vi "Build Tree.vi"(5 "Defer Updates (T)":bool=TRUE, 7 "Tree":refnum<vi>, 8 "error in (no error)":errorcluster, 11 "Tree Map in":refnum<class "Tree Map.lvclass">) -> (0 "error out":errorcluster, 3 "Tree Map out":refnum<class "Tree Map.lvclass">)   [LabVIEW 2020, in "Tree Map.lvlib" / "Tree Map.lvclass"]
uses:
  Tree Map.lvclass
  Tree Map.lvclass/Tree Map.ctl
  Tree Map.lvlib
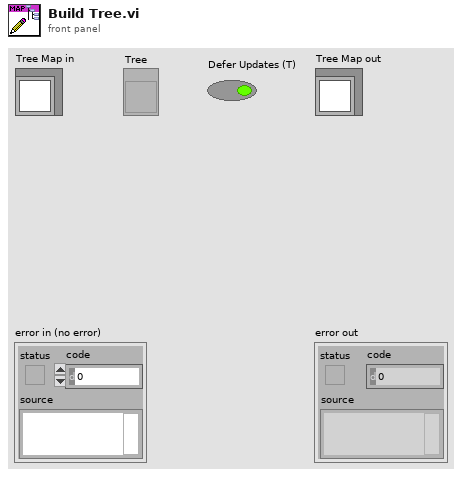
[diagram p1: front panel]
types:
  T1 = typedef "LVNodeAndColumnTypeDef.ctl" = cluster{"Node":string, "Column":i32}
  T2 = typedef "Tree Map.lvlib/Tree Map.lvclass/Tree Entry.ctl" = cluster{"Hierarchy":string[], "Name":string, "Columns":string[], "Leaf":bool, "Extra":T3}
  T3 = typedef "Tree Map.lvlib/Tree Map.lvclass/Extra Entry Info.ctl" = cluster{"BG Color":u32, "Symbol":i32}
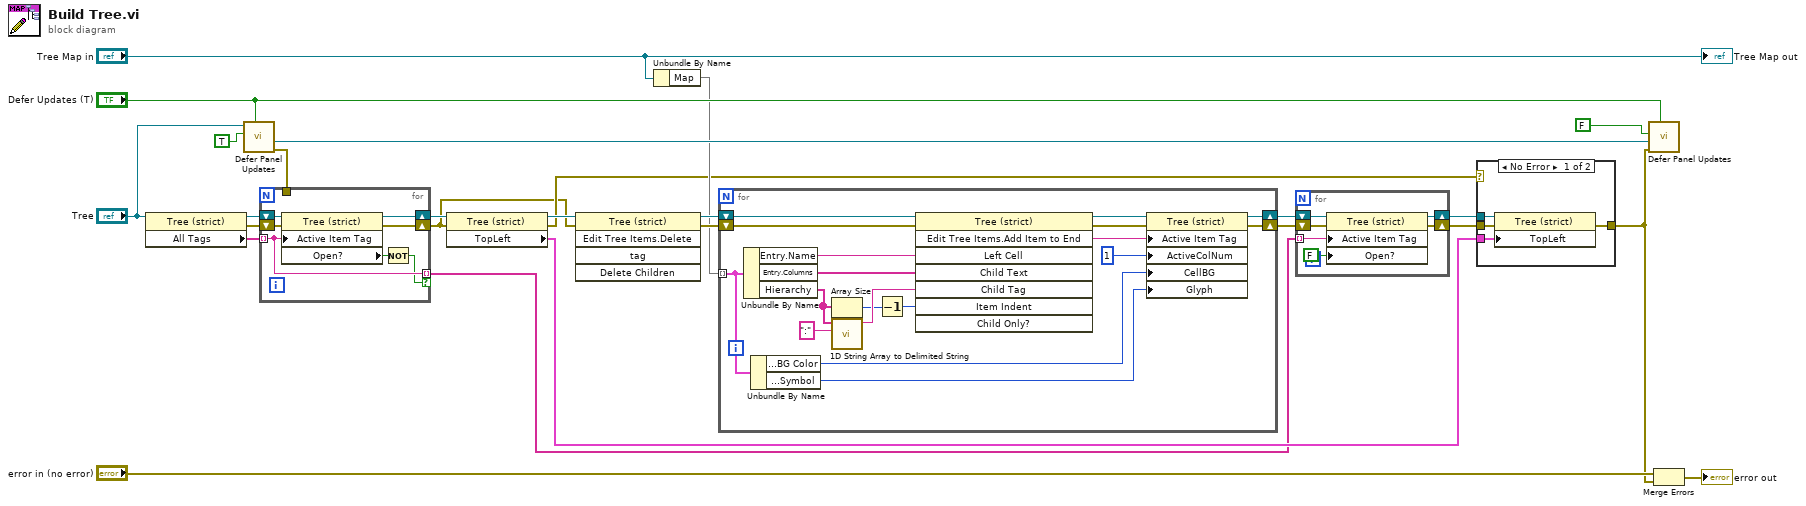
[diagram p0: block diagram]
diagram:
  n1 = property class="Tree (strict)"(reference="Tree") -> (reference out=w20:refnum<vi>, error out=w7:errorcluster, "All Tags"=w21:string[])  [unwired: 1 in]
  n2 = call "Defer Panel Updates.vi"("Set Defer (T)"="Defer Updates (T)", "Defer"=TRUE, "Tree (Front Panel)"="Tree") -> ("error out"=w8:errorcluster, "Front Panel"=w12:refnum<vi>)  [unwired: 7 in]
  n3 = for {
    tunnel: w21 -> [w31] mode=indexing
    shift-right: [w29] -> w19
    shift-left: w20 -> [w33]
    tunnel: [w31] -> w18 mode=indexing if=w30
    tunnel: w8 -> [_]
    shift-right: [w27] -> w1
    shift-left: w7 -> [w28]
    n4 = property class="Tree (strict)"(reference=w33, error in=w28, "Active Item Tag"=w31) -> (reference out=w29:refnum<vi>, error out=w27:errorcluster, "Open?"=w32:bool)
    n5 = Not(x=w32) -> (.not. x?=w30:bool)
  }
  n6 = property class="Tree (strict)"(reference=w19, error in=w1) -> (reference out=w23:refnum<vi>, error out=w2:errorcluster, "TopLeft"=w22:T1)
  n7 = invoke class="Tree (strict)" method="Edit Tree Items.Delete"(reference=w23, error in=w1) -> (reference out=w24:refnum<vi>, error out=w26:errorcluster)  [unwired: 3 in, 3 out]
  n8 = Unbundle By Name("Tree Map in") -> ("Map"=w9:map{string[], T2})
  n9 = for {
    shift-right: [w37] -> w16
    shift-left: w24 -> [w51]
    tunnel: w9 -> [w42] mode=indexing
    shift-right: [w36] -> w6
    shift-left: w26 -> [w44]
    n10 = Unbundle By Name(w42) -> ("Entry.Name"=w45:string, "Entry.Columns"=w46:string[], "Hierarchy"=w43:string[])
    n11 = Unbundle By Name(w42) -> ("Entry.Extra.BG Color"=w35:u32, "Entry.Extra.Symbol"=w34:i32)
    n12 = Array Size(array=w43) -> (size(s)=w48:i32)
    n13 = call <vilib>:"1D String Array to Delimited String.vi"("delimiter"=":", "string array"=w43) -> ("delimited string"=w49:string)  [unwired: 9 in]
    n14 = Decrement(x=w48) -> (x-1=w47:i32)
    n15 = invoke class="Tree (strict)" method="Edit Tree Items.Add Item to End"(reference=w51, error in=w44, "Left Cell"=w45, "Child Text"=w46, "Child Tag"=w49, "Item Indent"=w47) -> (reference out=w41:refnum<vi>, error out=w40:errorcluster, "Edit Tree Items:Add Item to End"=w39:string)  [unwired: 2 in, 5 out]
    n16 = property class="Tree (strict)"(reference=w41, error in=w40, "Active Item Tag"=w39, "ActiveColNum"=1 ("Active Cell:Active Column Number"), "CellBG"=w35, "Glyph"=w34) -> (reference out=w37:refnum<vi>, error out=w36:errorcluster)
  }
  n17 = for {
    shift-right: [w56] -> w17
    shift-left: w16 -> [w57]
    tunnel: w18 -> [w54] mode=indexing
    shift-right: [w52] -> w5
    shift-left: w6 -> [w53]
    n18 = property class="Tree (strict)"(reference=w57, error in=w53, "Active Item Tag"=w54, "Open?"=FALSE ("Active Item:Open?")) -> (reference out=w56:refnum<vi>, error out=w52:errorcluster)
  }
  n19 = case shown="No Error" w2 {
    tunnel: w22 -> [w61 _]
    tunnel: w17 -> [w60 _]
    tunnel: w5 -> [w59 w62]
    tunnel: [w58 w62] -> w3
    frame No Error {
      n20 = property class="Tree (strict)"(reference=w60, error in=w59, "TopLeft"=w61) -> (error out=w58:errorcluster)  [unwired: 1 out]
    }
    frame Error {
    }
  }
  n21 = call "Defer Panel Updates.vi"("Set Defer (T)"="Defer Updates (T)", "error in (no error)"=w3, "Front Panel (Lookup)"=w12, "Defer"=FALSE ("Defer Panel Updates")) -> ()  [unwired: 6 in, 2 out]
  n22 = Merge Errors("error in (no error)", w3) -> (→"error out":errorcluster)
  "Tree Map out" <- "Tree Map in"
